vi "5RobotsSkill.vi"(5 "Eliminate":T1, 6 "id":i32, 7 "5Positions":dbl[][](array[numeric]), 8 "error in (no error)":errorcluster, 9 "Robot In":refnum<class "Robot.lvclass">, 10 "Game in":refnum<class "Game.lvclass">, 11 "5RobotsSkill in":refnum<class "5RobotsSkill.lvclass">) -> (0 "error out":errorcluster, 2 "Robot out":refnum<class "Robot.lvclass">, 3 "5RobotsSkill out":refnum<class "5RobotsSkill.lvclass">)   [LabVIEW 2020, in "5RobotsSkill.lvclass"]
uses:
  5RobotsSkill.lvclass
  Game_class/Game.lvclass
  Robot_class/Robot.lvclass
  Ally_class/EliminateEnum.ctl
  Utilities_class/Utilities.lvclass
  Game_class/Game.lvclass/Game.ctl
  Referee_class/Referee.lvclass/Referee.ctl
  Team_class/Team.lvclass/Team.ctl
  Robot_class/Robot.lvclass/Robot.ctl
  d6476285-48f6-47f5-bd76-da5b47b6f033.vi
  b4841ea0-fdbc-4f48-b81d-56e09d8e2016.vi
  0d12ad11-68e3-46b2-a192-4422364186e5.vi
  6660b6ff-d865-414d-86e9-5587d6df92b5.vi
  8726d1a9-8fa9-45be-ba09-7ecc15164713.vi
  Robot_class/Read id.vi
  3b771abe-fd57-4fcc-a3fe-9fcf721aac13.vi
  Team_class/Read RobotRef.vi
  Game_class/Read BallRef.vi
  Game_class/Read Referee.vi
  Referee_class/Read our_goalie_id.vi
  Game_class/Read AllyRef.vi
  Robot_class/Write dest_x.vi
  Robot_class/Write dest_y.vi
  Robot_class/Write dest_orientation.vi
  Robot_class/Write keepDest.vi
  <vilib>/Array/Sort 2D Array - Pop Stack.vi
  <vilib>/Array/Sort 2D Array - Push Stack.vi
  d6476285-48f6-47f5-bd76-da5b47b6f033.vi/269d4b3b-47f5-49e3-8884-44851e4dd9d5.vi
  d6476285-48f6-47f5-bd76-da5b47b6f033.vi/6d99389c-673d-4efb-bf33-19b32bcf4cf8.vi
  b4841ea0-fdbc-4f48-b81d-56e09d8e2016.vi/269d4b3b-47f5-49e3-8884-44851e4dd9d5.vi
  b4841ea0-fdbc-4f48-b81d-56e09d8e2016.vi/6d99389c-673d-4efb-bf33-19b32bcf4cf8.vi
  0d12ad11-68e3-46b2-a192-4422364186e5.vi/269d4b3b-47f5-49e3-8884-44851e4dd9d5.vi
  0d12ad11-68e3-46b2-a192-4422364186e5.vi/6d99389c-673d-4efb-bf33-19b32bcf4cf8.vi
  6660b6ff-d865-414d-86e9-5587d6df92b5.vi/269d4b3b-47f5-49e3-8884-44851e4dd9d5.vi
  6660b6ff-d865-414d-86e9-5587d6df92b5.vi/6d99389c-673d-4efb-bf33-19b32bcf4cf8.vi
  8726d1a9-8fa9-45be-ba09-7ecc15164713.vi/269d4b3b-47f5-49e3-8884-44851e4dd9d5.vi
  8726d1a9-8fa9-45be-ba09-7ecc15164713.vi/6d99389c-673d-4efb-bf33-19b32bcf4cf8.vi
  Ally_class/Ally.lvclass
  C:/Users/anton/Desktop/RoboIME/SSL_COMP/SSL_AI/Team_class/Team.lvclass
  Ball_class/Ball.lvclass
  Referee_class/Referee.lvclass
  <vilib>/Comparison/Less/Less Functor/Less Functor.lvclass
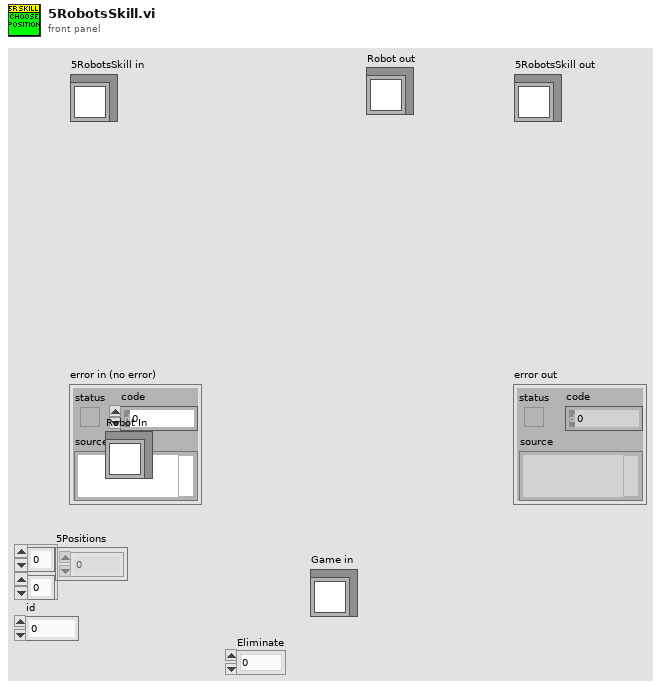
[diagram p1: front panel]
types:
  T1 = typedef "EliminateEnum.ctl" = enum16{"0", "1", "2"}
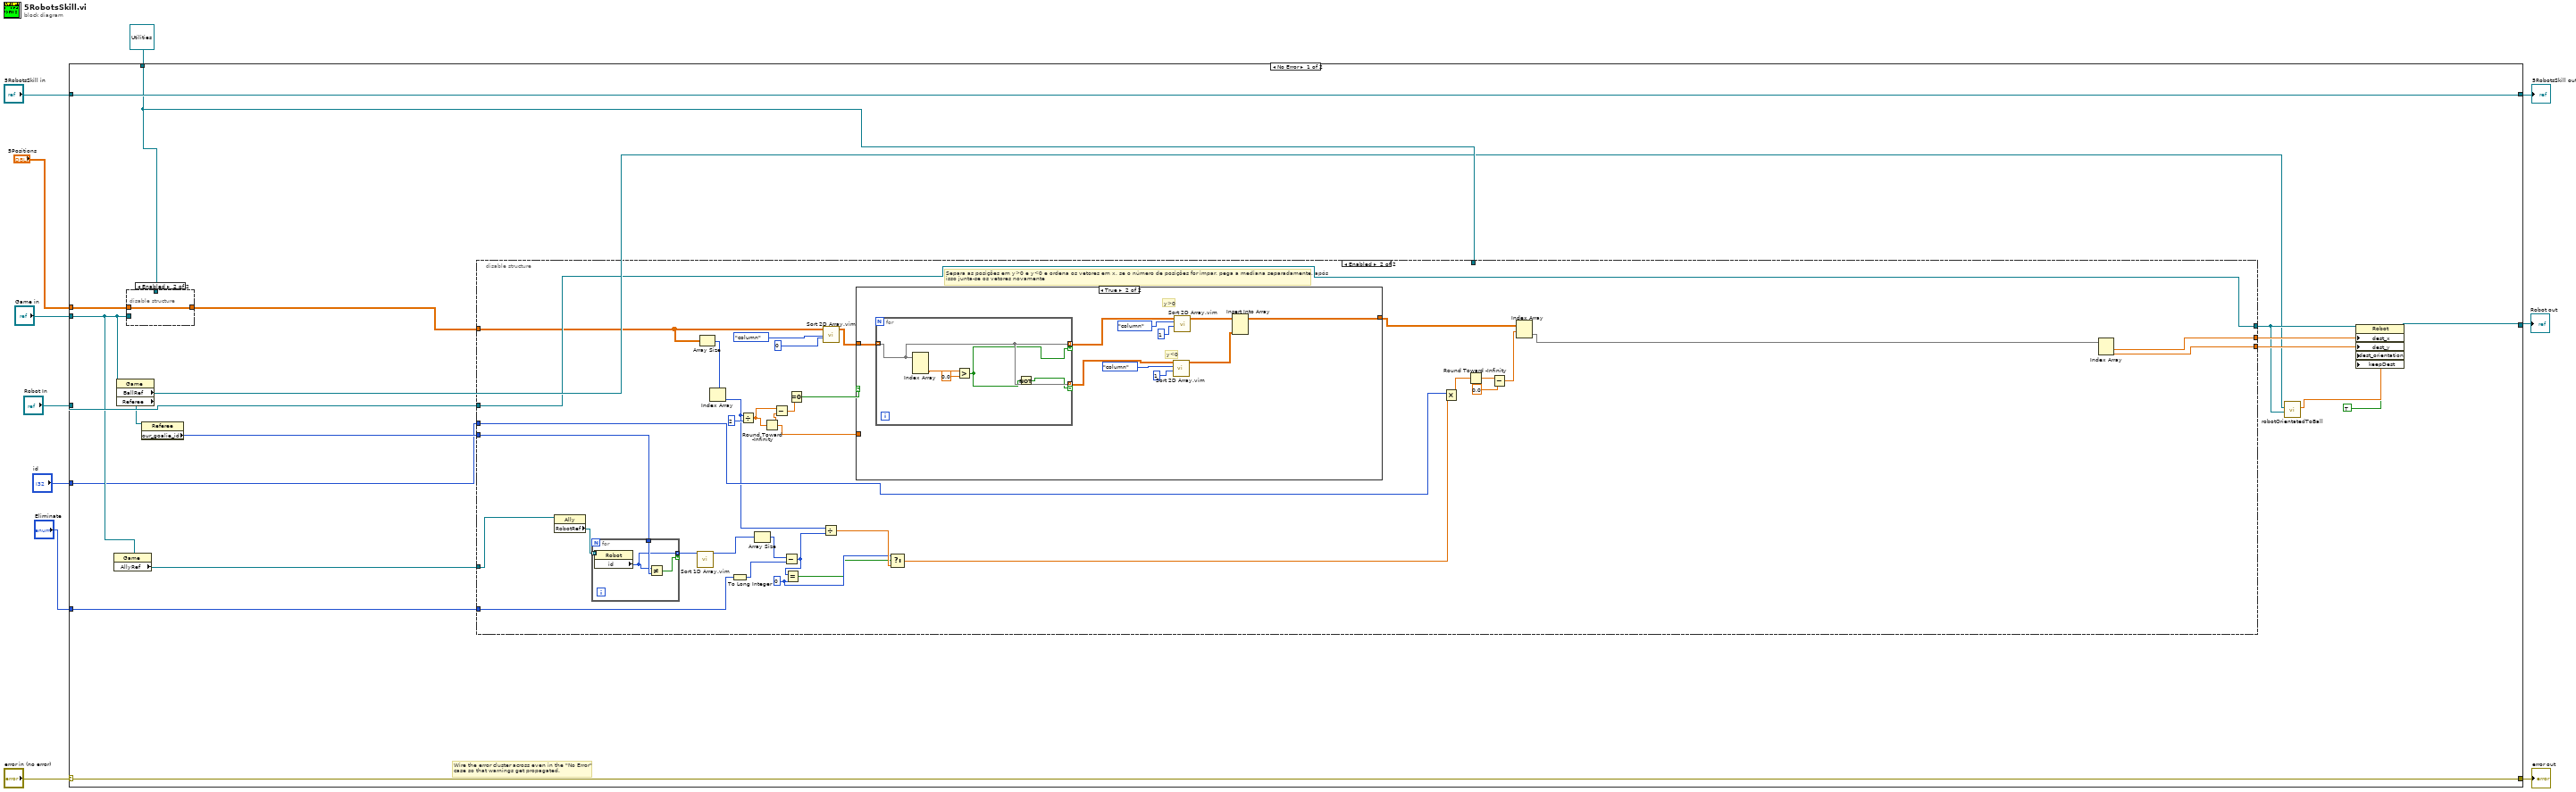
[diagram p0: block diagram]
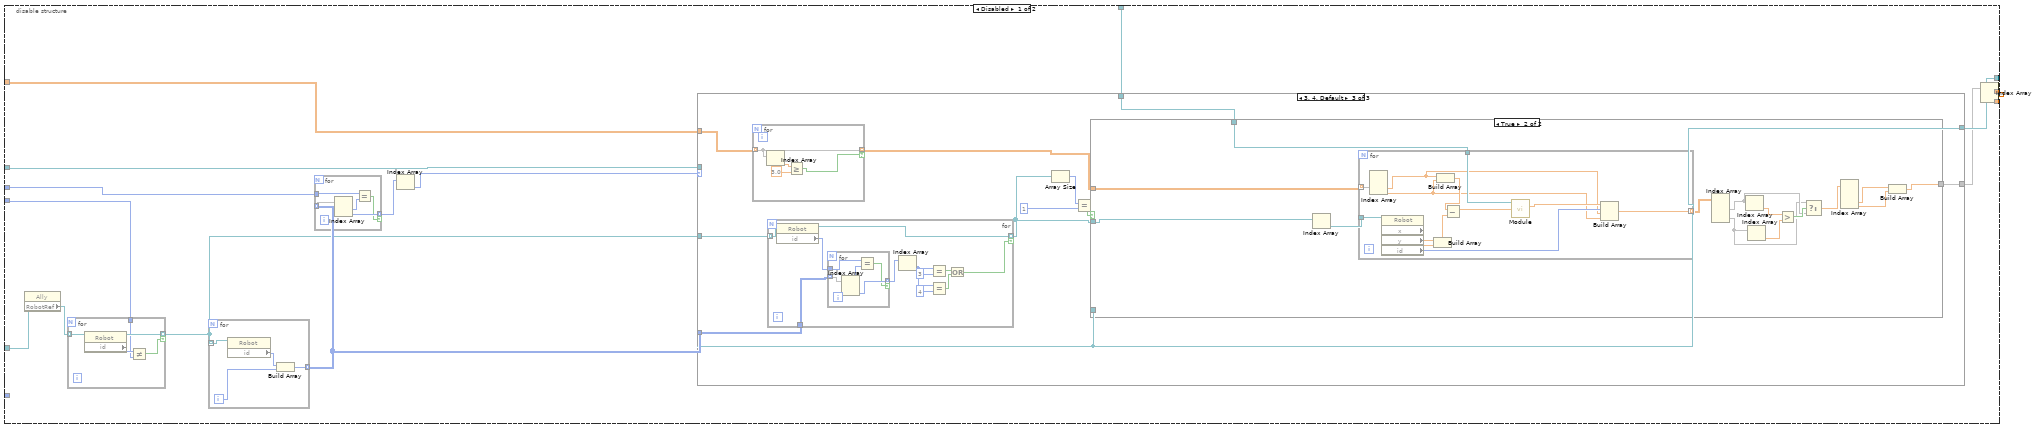
[diagram p2: hidden frame]
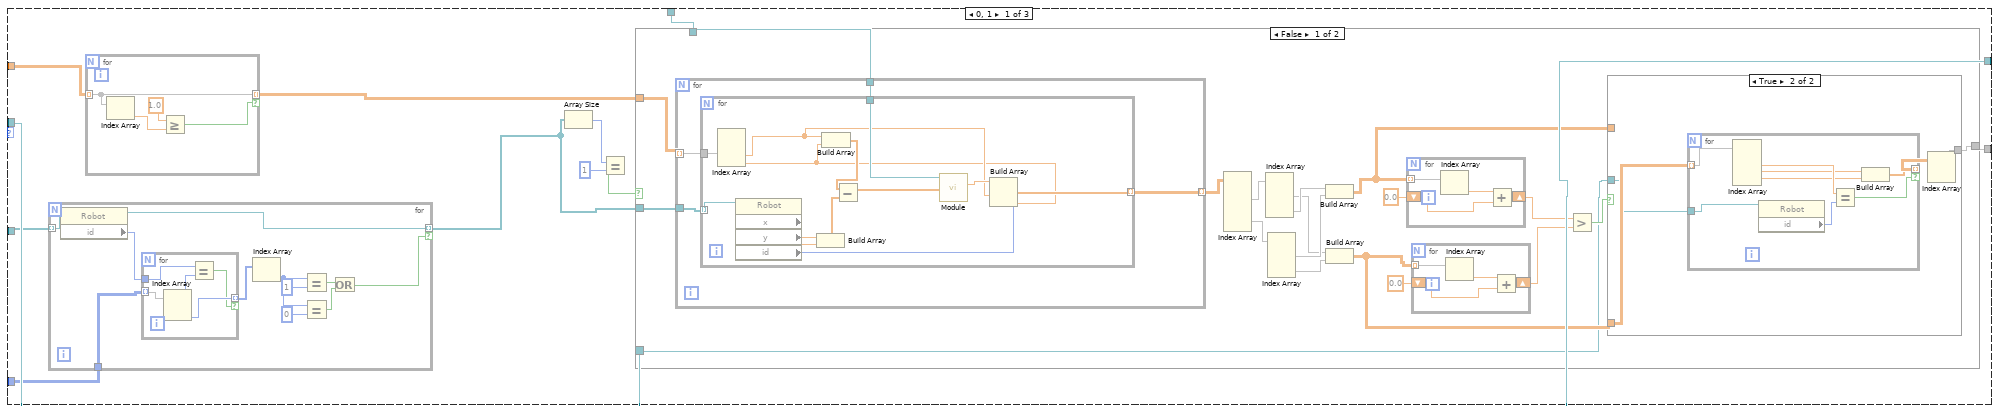
[diagram p3: hidden frame]
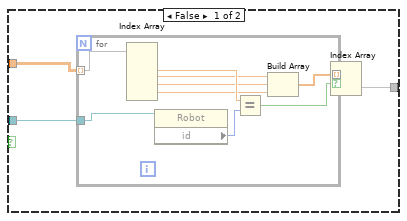
[diagram p4: hidden frame]
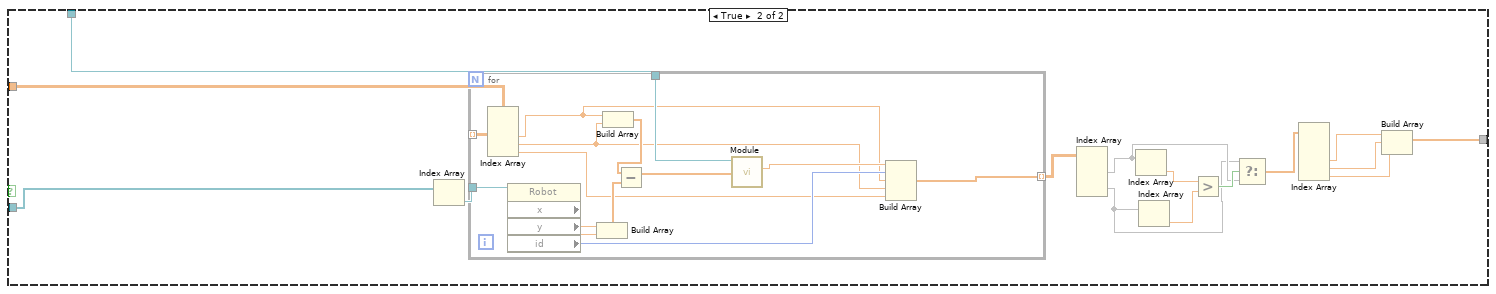
[diagram p5: hidden frame]
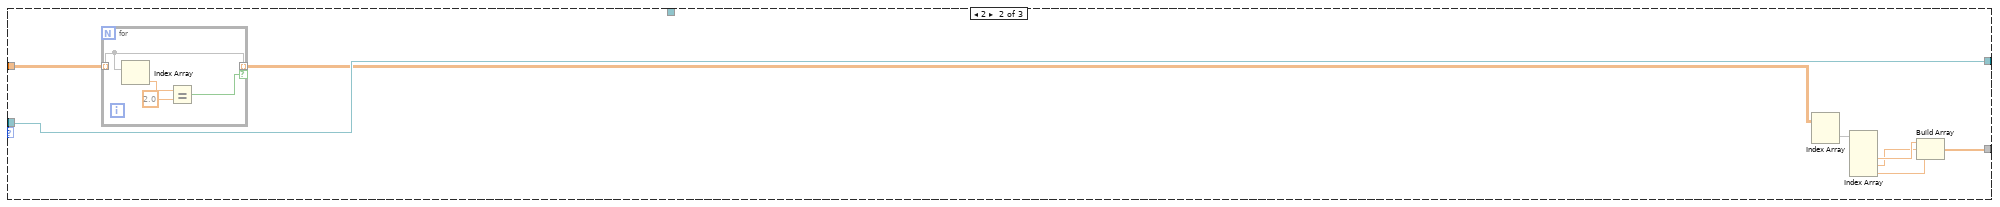
[diagram p6: hidden frame]
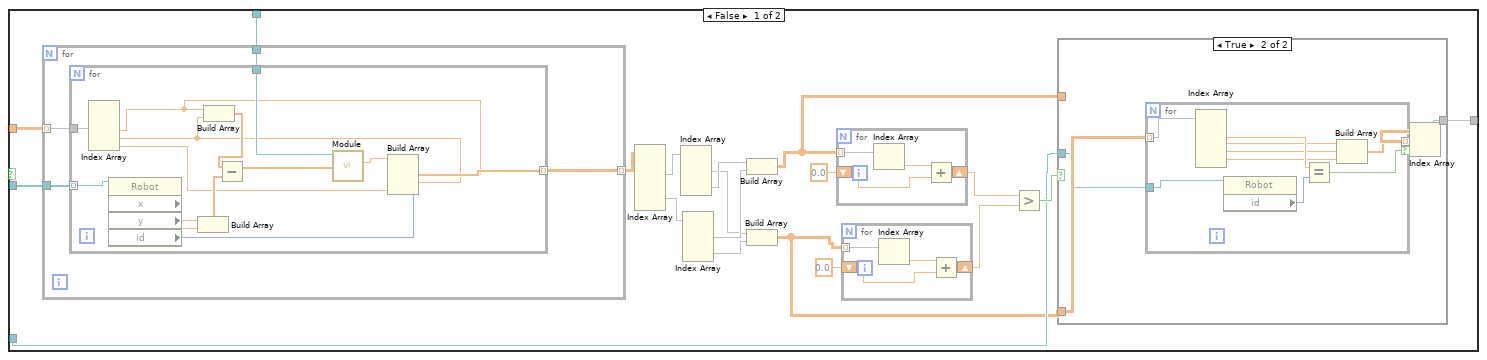
[diagram p7: hidden frame]
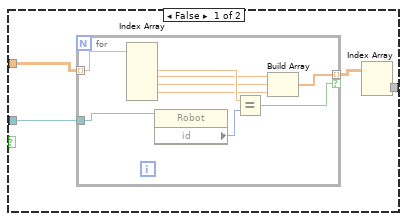
[diagram p8: hidden frame]
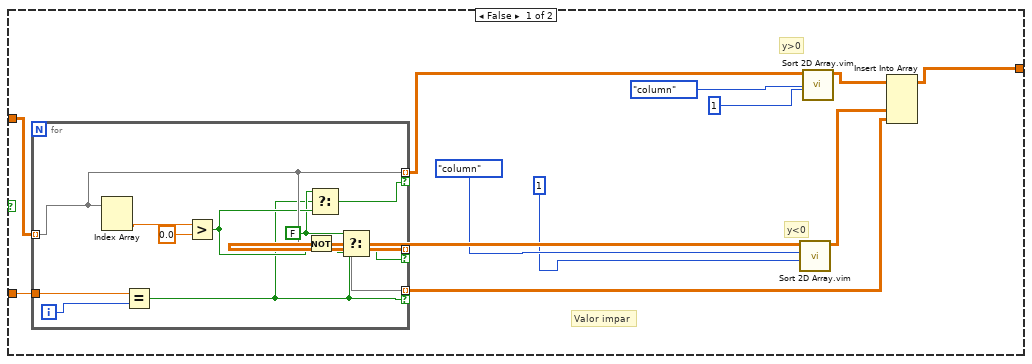
[diagram p9: hidden frame]
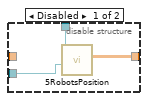
[diagram p10: hidden frame]
diagram:
  n1 = case shown="No Error" "error in (no error)" {
    selector: "error in (no error)" -> [w29 w412]
    tunnel: [w29 w412] -> w10
    tunnel: [w30 w411] -> w8
    tunnel: "5RobotsSkill in" -> [w30 w411]
    tunnel: refnum<class "Utilities.lvclass"> refnum ("Utilities in") -> [w27 _]
    tunnel: "Game in" -> [w21 _]
    tunnel: "Robot In" -> [w28 w410]
    tunnel: [w26 w410] -> w4
    tunnel: "5Positions" -> [w19 _]
    tunnel: "id" -> [w13 _]
    tunnel: "Eliminate" -> [w12 _]
    frame No Error {
      # "Wire the error cluster across even in the \"No Error\"\ncase so that warnings get propagated."
      n2 = property class="Game"(reference=w21) -> ("AllyRef"=w17:refnum<class "Ally.lvclass">)  [unwired: 1 in, 2 out]
      n3 = property class="Game"(reference=w21) -> ("BallRef"=w20:refnum<class "Ball.lvclass">, "Referee"=w16:refnum<class "Referee.lvclass">)  [unwired: 1 in, 2 out]
      n4 = disable-structure shown="Enabled" {
        disable-tunnel: [w408 w409] -> w14
        disable-tunnel: w27 -> [w407 _]
        disable-tunnel: w21 -> [w406 _]
        disable-tunnel: w19 -> [_ w409]
        frame Disabled {
          n5 = call-dynamic "5RobotsPosition.vi"("Game"=w406, "Utilities in"=w407) -> ("5Positions"=w408:dbl[][])  [unwired: 7 in, 2 out]
        }
        frame Enabled {
        }
      }
      n6 = property class="Referee"(reference=w16) -> ("our_goalie_id"=w15:i32)  [unwired: 1 in, 2 out]
      n7 = disable-structure shown="Enabled" {
        disable-tunnel: w28 -> [w45 w344]
        disable-tunnel: w27 -> [w44 _]
        disable-tunnel: [w43 w338] -> w24
        disable-tunnel: [w42 w343] -> w23
        disable-tunnel: [w41 w344] -> w22
        disable-tunnel: w17 -> [w40 w362]
        disable-tunnel: w13 -> [w38 w351]
        disable-tunnel: w15 -> [w33 w361]
        disable-tunnel: w14 -> [w32 w340]
        disable-tunnel: w12 -> [_ w333]
        frame Disabled {
          n8 = property class="Ally"(reference=w40) -> ("RobotRef"=w34:refnum<class "Robot.lvclass">[])  [unwired: 1 in, 2 out]
          n9 = for {
            tunnel: w34 -> [w320] mode=indexing
            tunnel: [w319] -> w31 mode=indexing if=w317
            tunnel: w33 -> [w316]
            n10 = property class="Robot"(reference=w320) -> (reference out=w319:refnum<class "Robot.lvclass">, "id"=w318:i32)  [unwired: 1 in, 1 out]
            n11 = Not Equal?(x=w318, y=w316) -> (x != y?=w317:bool)
          }
          n12 = for {
            tunnel: w31 -> [w329] mode=indexing
            tunnel: [w327] -> w35 mode=indexing
            i -> [w326]
            n13 = property class="Robot"(reference=w329) -> ("id"=w328:i32)  [unwired: 1 in, 2 out]
            n14 = Build Array(w328, w326) -> (w327:i32[])
          }
          n15 = for {
            tunnel: w38 -> [w322]
            tunnel: w35 -> [w325] mode=indexing
            tunnel: [w324] -> w36 mode=indexing if=w321
            n16 = Index Array(array=w325) -> (element #1=w323:i32, element #2=w324:i32)  [unwired: 2 in]
            n17 = Equal?(x=w322, y=w323) -> (x = y?=w321:bool)
          }
          n18 = Index Array(array=w36) -> (element=w37:i32)  [unwired: 1 in]
          n19 = case shown="3, 4, Default" w37 {
            tunnel: w44 -> [w56 _ w196]
            tunnel: w45 -> [w54 w181 w194]
            tunnel: w32 -> [w50 w182 w197]
            tunnel: [w55 w176 w195] -> w39
            tunnel: [w54 w181 w194] -> w41
            tunnel: w31 -> [w48 _ w188]
            tunnel: w35 -> [w47 _ w187]
            frame 0, 1 {
              n20 = for {
                tunnel: [w165] -> w46 mode=indexing if=w155
                tunnel: w48 -> [w164] mode=indexing
                tunnel: w47 -> [w162]
                n21 = property class="Robot"(reference=w164) -> (reference out=w165:refnum<class "Robot.lvclass">, "id"=w163:i32)  [unwired: 1 in, 1 out]
                n22 = for {
                  tunnel: w163 -> [w169]
                  tunnel: w162 -> [w170] mode=indexing
                  tunnel: [w167] -> w161 mode=indexing if=w166
                  n23 = Index Array(array=w170) -> (element #1=w168:i32, element #2=w167:i32)  [unwired: 2 in]
                  n24 = Equal?(x=w169, y=w168) -> (x = y?=w166:bool)
                }
                n25 = Index Array(array=w161) -> (element=w160:i32)  [unwired: 1 in]
                n26 = Equal?(x=w160, y=1) -> (x = y?=w157:bool)
                n27 = Equal?(x=w160, y=0) -> (x = y?=w156:bool)
                n28 = Or(x=w157, y=w156) -> (x .or. y?=w155:bool)
              }
              n29 = for {
                tunnel: w50 -> [w174] mode=indexing
                tunnel: [w174] -> w49 mode=indexing if=w173
                n30 = Index Array(array=w174) -> (element=w171:dbl)  [unwired: 1 in]
                n31 = Greater Or Equal?(x=1.0 ("y"), y=w171) -> (x >= y?=w173:bool)
              }
              n32 = Array Size(array=w46) -> (size(s)=w51:i32)
              n33 = Equal?(x=w51, y=1) -> (x = y?=w53:bool)
              n34 = case shown="False" w53 {
                tunnel: w46 -> [w75 w138]
                tunnel: w56 -> [w74 w136]
                tunnel: w49 -> [w73 w139]
                tunnel: [w57 w140] -> w55
                tunnel: w54 -> [w58 _]
                frame False {
                  n35 = for {
                    tunnel: w75 -> [w112]
                    tunnel: w74 -> [w111]
                    tunnel: w73 -> [w110] mode=indexing
                    tunnel: [w109] -> w59 mode=indexing
                    n36 = for {
                      tunnel: w112 -> [w125] mode=indexing
                      tunnel: w110 -> [w117]
                      tunnel: w111 -> [w120]
                      tunnel: [w119] -> w109 mode=indexing
                      n37 = Index Array(array=w117) -> (element #2=w114:dbl, element #3=w113:dbl)  [unwired: 3 in, 1 out]
                      n38 = property class="Robot"(reference=w125) -> ("x"=w124:dbl, "y"=w123:dbl, "id"=w116:i32)  [unwired: 1 in, 2 out]
                      n39 = Build Array(w124, w123) -> (w122:dbl[])
                      n40 = Build Array(w114, w113) -> (w115:dbl[])
                      n41 = Subtract(x=w115, y=w122) -> (x-y=w121:dbl[])
                      n42 = call "Module.vi"("2D vector"=w121, "Utilities in"=w120) -> ("Modulo"=w118:dbl)  [unwired: 7 in, 2 out]
                      n43 = Build Array(w118, w116, w114, w113) -> (w119:dbl[])
                    }
                  }
                  n44 = Index Array(array=w59) -> (element #1=w67:dbl[][], element #2=w66:dbl[][])  [unwired: 6 in]
                  n45 = Index Array(array=w67) -> (element #1=w63:dbl[], element #2=w64:dbl[])  [unwired: 4 in]
                  n46 = Index Array(array=w66) -> (element #1=w65:dbl[], element #2=w62:dbl[])  [unwired: 4 in]
                  n47 = Build Array(w64, w65) -> (w60:dbl[][])
                  n48 = Build Array(w63, w62) -> (w61:dbl[][])
                  n49 = for {
                    tunnel: w60 -> [w108] mode=indexing
                    shift-right: [w106] -> w70
                    shift-left: 0.0 -> [w105]
                    n50 = Index Array(array=w108) -> (element=w107:dbl)  [unwired: 1 in]
                    n51 = Add(x=w107, y=w105) -> (x+y=w106:dbl)
                  }
                  n52 = for {
                    tunnel: w61 -> [w104] mode=indexing
                    shift-right: [w102] -> w69
                    shift-left: 0.0 -> [w101]
                    n53 = Index Array(array=w104) -> (element=w103:dbl)  [unwired: 1 in]
                    n54 = Add(x=w103, y=w101) -> (x+y=w102:dbl)
                  }
                  n55 = Greater?(x=w70, y=w69) -> (0:w68:bool)
                  n56 = case shown="True" w68 {
                    tunnel: w60 -> [w79 _]
                    tunnel: w61 -> [_ w90]
                    tunnel: w58 -> [w78 w89]
                    tunnel: [w76 w91] -> w57
                    frame False {
                      n57 = for {
                        tunnel: w79 -> [w87] mode=indexing
                        tunnel: w78 -> [w88]
                        tunnel: [w81] -> w77 mode=indexing if=w80
                        n58 = Index Array(array=w87) -> (element #2=w85:dbl, element #3=w84:dbl, element #4=w83:dbl, element #5=w82:dbl)  [unwired: 5 in, 1 out]
                        n59 = property class="Robot"(reference=w88) -> ("id"=w86:i32)  [unwired: 1 in, 2 out]
                        n60 = Equal?(x=w85, y=w86) -> (x = y?=w80:bool)
                        n61 = Build Array(w84, w83, w82) -> (w81:dbl[])
                      }
                      n62 = Index Array(array=w77) -> (element=w76:dbl[])  [unwired: 2 in]
                    }
                    frame True {
                      n63 = for {
                        tunnel: w90 -> [w99] mode=indexing
                        tunnel: w89 -> [w100]
                        tunnel: [w94] -> w92 mode=indexing if=w93
                        n64 = Index Array(array=w99) -> (element #2=w97:dbl, element #3=w96:dbl, element #4=w95:dbl)  [unwired: 4 in, 1 out]
                        n65 = property class="Robot"(reference=w100) -> ("id"=w98:i32)  [unwired: 1 in, 2 out]
                        n66 = Equal?(x=w97, y=w98) -> (x = y?=w93:bool)
                        n67 = Build Array(w96, w95) -> (w94:dbl[])
                      }
                      n68 = Index Array(array=w92) -> (element=w91:dbl[])  [unwired: 2 in]
                    }
                  }
                }
                frame True {
                  n69 = Index Array(array=w138) -> (element=w137:refnum<class "Robot.lvclass">)  [unwired: 1 in]
                  n70 = for {
                    tunnel: w139 -> [w147] mode=indexing
                    tunnel: w136 -> [w150]
                    tunnel: [w149] -> w135 mode=indexing
                    tunnel: w137 -> [w141]
                    n71 = Index Array(array=w147) -> (element #2=w144:dbl, element #3=w143:dbl, element #4=w142:dbl)  [unwired: 4 in, 1 out]
                    n72 = property class="Robot"(reference=w141) -> ("x"=w154:dbl, "y"=w153:dbl, "id"=w146:i32)  [unwired: 1 in, 2 out]
                    n73 = Build Array(w154, w153) -> (w152:dbl[])
                    n74 = Build Array(w144, w143) -> (w145:dbl[])
                    n75 = Subtract(x=w145, y=w152) -> (x-y=w151:dbl[])
                    n76 = call "Module.vi"("2D vector"=w151, "Utilities in"=w150) -> ("Modulo"=w148:dbl)  [unwired: 7 in, 2 out]
                    n77 = Build Array(w148, w146, w144, w143, w142) -> (w149:dbl[])
                  }
                  n78 = Index Array(array=w135) -> (element #1=w131:dbl[], element #2=w130:dbl[])  [unwired: 4 in]
                  n79 = Index Array(array=w131) -> (element=w134:dbl)  [unwired: 1 in]
                  n80 = Index Array(array=w130) -> (element=w133:dbl)  [unwired: 1 in]
                  n81 = Greater?(x=w134, y=w133) -> (0:w132:bool)
                  n82 = Select(t=w130, s=w132, f=w131) -> (s? t:f=w129:dbl[])
                  n83 = Index Array(array=w129) -> (element #3=w128:dbl, element #4=w127:dbl, element #5=w126:dbl)  [unwired: 5 in, 2 out]
                  n84 = Build Array(w128, w127, w126) -> (w140:dbl[])
                }
              }
            }
            frame 2 {
              n85 = for {
                tunnel: w182 -> [w185] mode=indexing
                tunnel: [w185] -> w175 mode=indexing if=w186
                n86 = Index Array(array=w185) -> (element=w184:dbl)  [unwired: 1 in]
                n87 = Equal?(x=w184, y=2.0) -> (x = y?=w186:bool)
              }
              n88 = Index Array(array=w175) -> (element=w180:dbl[])  [unwired: 2 in]
              n89 = Index Array(array=w180) -> (element #2=w179:dbl, element #3=w178:dbl, element #4=w177:dbl)  [unwired: 4 in, 1 out]
              n90 = Build Array(w179, w178, w177) -> (w176:dbl[])
            }
            frame 3, 4, Default {
              n91 = for {
                tunnel: w197 -> [w315] mode=indexing
                tunnel: [w315] -> w191 mode=indexing if=w314
                n92 = Index Array(array=w315) -> (element=w312:dbl)  [unwired: 1 in]
                n93 = Greater Or Equal?(x=w312, y=3.0) -> (x >= y?=w314:bool)
              }
              n94 = for {
                tunnel: [w306] -> w189 mode=indexing if=w296
                tunnel: w188 -> [w305] mode=indexing
                tunnel: w187 -> [w303]
                n95 = property class="Robot"(reference=w305) -> (reference out=w306:refnum<class "Robot.lvclass">, "id"=w304:i32)  [unwired: 1 in, 1 out]
                n96 = for {
                  tunnel: w304 -> [w310]
                  tunnel: w303 -> [w311] mode=indexing
                  tunnel: [w308] -> w302 mode=indexing if=w307
                  n97 = Index Array(array=w311) -> (element #1=w309:i32, element #2=w308:i32)  [unwired: 2 in]
                  n98 = Equal?(x=w310, y=w309) -> (x = y?=w307:bool)
                }
                n99 = Index Array(array=w302) -> (element=w301:i32)  [unwired: 1 in]
                n100 = Equal?(x=w301, y=3) -> (x = y?=w298:bool)
                n101 = Equal?(x=w301, y=4) -> (x = y?=w297:bool)
                n102 = Or(x=w298, y=w297) -> (x .or. y?=w296:bool)
              }
              n103 = Array Size(array=w189) -> (size(s)=w190:i32)
              n104 = Equal?(x=w190, y=1) -> (x = y?=w192:bool)
              n105 = case shown="True" w192 {
                tunnel: w196 -> [w216 w270]
                tunnel: w191 -> [w215 w271]
                tunnel: [w208 w272] -> w195
                tunnel: w194 -> [w207 _]
                tunnel: w189 -> [w198 w269]
                frame False {
                  n106 = for {
                    tunnel: w216 -> [w254]
                    tunnel: w215 -> [w253] mode=indexing
                    tunnel: [w252] -> w214 mode=indexing
                    tunnel: w198 -> [w251]
                    n107 = for {
                      tunnel: w253 -> [w261]
                      tunnel: w254 -> [w264]
                      tunnel: [w263] -> w252 mode=indexing
                      tunnel: w251 -> [w255] mode=indexing
                      n108 = Index Array(array=w261) -> (element #2=w258:dbl, element #3=w257:dbl, element #4=w256:dbl)  [unwired: 4 in, 1 out]
                      n109 = property class="Robot"(reference=w255) -> ("x"=w268:dbl, "y"=w267:dbl, "id"=w260:i32)  [unwired: 1 in, 2 out]
                      n110 = Build Array(w268, w267) -> (w266:dbl[])
                      n111 = Build Array(w258, w257) -> (w259:dbl[])
                      n112 = Subtract(x=w259, y=w266) -> (x-y=w265:dbl[])
                      n113 = call "Module.vi"("2D vector"=w265, "Utilities in"=w264) -> ("Modulo"=w262:dbl)  [unwired: 7 in, 2 out]
                      n114 = Build Array(w262, w260, w258, w257, w256) -> (w263:dbl[])
                    }
                  }
                  n115 = Index Array(array=w214) -> (element #1=w206:dbl[][], element #2=w205:dbl[][])  [unwired: 6 in]
                  n116 = Index Array(array=w206) -> (element #1=w202:dbl[], element #2=w203:dbl[])  [unwired: 4 in]
                  n117 = Index Array(array=w205) -> (element #1=w204:dbl[], element #2=w201:dbl[])  [unwired: 4 in]
                  n118 = Build Array(w203, w204) -> (w199:dbl[][])
                  n119 = Build Array(w202, w201) -> (w200:dbl[][])
                  n120 = for {
                    tunnel: w199 -> [w250] mode=indexing
                    shift-right: [w248] -> w211
                    shift-left: 0.0 -> [w247]
                    n121 = Index Array(array=w250) -> (element=w249:dbl)  [unwired: 1 in]
                    n122 = Add(x=w249, y=w247) -> (x+y=w248:dbl)
                  }
                  n123 = for {
                    tunnel: w200 -> [w246] mode=indexing
                    shift-right: [w244] -> w210
                    shift-left: 0.0 -> [w243]
                    n124 = Index Array(array=w246) -> (element=w245:dbl)  [unwired: 1 in]
                    n125 = Add(x=w245, y=w243) -> (x+y=w244:dbl)
                  }
                  n126 = Greater?(x=w211, y=w210) -> (0:w209:bool)
                  n127 = case shown="True" w209 {
                    tunnel: w199 -> [w220 _]
                    tunnel: w200 -> [_ w231]
                    tunnel: w207 -> [w219 w230]
                    tunnel: [w217 w232] -> w208
                    frame False {
                      n128 = for {
                        tunnel: w220 -> [w228] mode=indexing
                        tunnel: w219 -> [w229]
                        tunnel: [w222] -> w218 mode=indexing if=w221
                        n129 = Index Array(array=w228) -> (element #2=w226:dbl, element #3=w225:dbl, element #4=w224:dbl, element #5=w223:dbl)  [unwired: 5 in, 1 out]
                        n130 = property class="Robot"(reference=w229) -> ("id"=w227:i32)  [unwired: 1 in, 2 out]
                        n131 = Equal?(x=w226, y=w227) -> (x = y?=w221:bool)
                        n132 = Build Array(w225, w224, w223) -> (w222:dbl[])
                      }
                      n133 = Index Array(array=w218) -> (element=w217:dbl[])  [unwired: 2 in]
                    }
                    frame True {
                      n134 = for {
                        tunnel: w231 -> [w241] mode=indexing
                        tunnel: w230 -> [w242]
                        tunnel: [w235] -> w233 mode=indexing if=w234
                        n135 = Index Array(array=w241) -> (element #2=w239:dbl, element #3=w238:dbl, element #4=w237:dbl, element #5=w236:dbl)  [unwired: 5 in, 1 out]
                        n136 = property class="Robot"(reference=w242) -> ("id"=w240:i32)  [unwired: 1 in, 2 out]
                        n137 = Equal?(x=w239, y=w240) -> (x = y?=w234:bool)
                        n138 = Build Array(w238, w237, w236) -> (w235:dbl[])
                      }
                      n139 = Index Array(array=w233) -> (element=w232:dbl[])  [unwired: 2 in]
                    }
                  }
                }
                frame True {
                  n140 = Index Array(array=w269) -> (element=w282:refnum<class "Robot.lvclass">)  [unwired: 1 in]
                  n141 = for {
                    tunnel: w271 -> [w288] mode=indexing
                    tunnel: w270 -> [w291]
                    tunnel: [w290] -> w281 mode=indexing
                    tunnel: w282 -> [w283]
                    n142 = Index Array(array=w288) -> (element #2=w285:dbl, element #3=w284:dbl)  [unwired: 3 in, 1 out]
                    n143 = property class="Robot"(reference=w283) -> ("x"=w295:dbl, "y"=w294:dbl, "id"=w287:i32)  [unwired: 1 in, 2 out]
                    n144 = Build Array(w295, w294) -> (w293:dbl[])
                    n145 = Build Array(w285, w284) -> (w286:dbl[])
                    n146 = Subtract(x=w286, y=w293) -> (x-y=w292:dbl[])
                    n147 = call "Module.vi"("2D vector"=w292, "Utilities in"=w291) -> ("Modulo"=w289:dbl)  [unwired: 7 in, 2 out]
                    n148 = Build Array(w289, w287, w285, w284) -> (w290:dbl[])
                  }
                  n149 = Index Array(array=w281) -> (element #1=w277:dbl[], element #2=w276:dbl[])  [unwired: 4 in]
                  n150 = Index Array(array=w277) -> (element=w280:dbl)  [unwired: 1 in]
                  n151 = Index Array(array=w276) -> (element=w279:dbl)  [unwired: 1 in]
                  n152 = Greater?(x=w280, y=w279) -> (0:w278:bool)
                  n153 = Select(t=w276, s=w278, f=w277) -> (s? t:f=w275:dbl[])
                  n154 = Index Array(array=w275) -> (element #3=w274:dbl, element #4=w273:dbl)  [unwired: 4 in, 2 out]
                  n155 = Build Array(w274, w273) -> (w272:dbl[])
                }
              }
            }
          }
          n156 = Index Array(array=w39) -> (element #1=w43:dbl, element #2=w42:dbl)  [unwired: 2 in]
        }
        frame Enabled {
          w336 = 0 ("y")
          # "Separa as posições em y>0 e y<0 e ordena os vetores em x, se o número de posições for impar, pega a mediana separadamente, após \nisso junta-se os vetores novamente"
          n157 = property class="Ally"(reference=w362) -> ("RobotRef"=w363:refnum<class "Robot.lvclass">[])  [unwired: 1 in, 2 out]
          n158 = for {
            tunnel: w363 -> [w405] mode=indexing
            tunnel: [w402] -> w360 mode=indexing if=w404
            tunnel: w361 -> [w403]
            n159 = property class="Robot"(reference=w405) -> ("id"=w402:i32)  [unwired: 1 in, 2 out]
            n160 = Not Equal?(x=w402, y=w403) -> (x != y?=w404:bool)
          }
          n161 = call "Sort 1D Array.vim"("unsorted array"=w360) -> ("sorted array"=w359:i32[])  [unwired: 10 in]
          n162 = Array Size(array=w340) -> (size(s)=w358:i32[])
          n163 = Index Array(array=w358) -> (element=w346:i32)  [unwired: 1 in]
          n164 = To Long Integer(number=w333) -> (32bit integer=w332:i32)
          n165 = Divide(x=w346, y=2) -> (x/y=w347:dbl)
          n166 = Array Size(array=w359) -> (size(s)=w334:i32)
          n167 = Round Toward -Infinity(1:w347) -> (0:w354:dbl)
          n168 = Subtract(x=w347, y=w354) -> (x-y=w355:dbl)
          n169 = Subtract(x=w334, y=w332) -> (x-y=w331:i32)
          n170 = Equal?(x=w331, y=w336) -> (x = y?=w330:bool)
          n171 = Equal To 0?(x=w355) -> (x = 0?=w356:bool)
          n172 = Divide(x=w346, y=w331) -> (x/y=w337:dbl)
          n173 = call "Sort 2D Array.vim"("index"=0, "dimension to index (column)"=enum16{"column", "row"}."column", "2D array"=w340) -> ("sorted 2D array"=w339:dbl[][])  [unwired: 7 in, 1 out]
          n174 = case shown="True" w356 {
            tunnel: w354 -> [w369 _]
            tunnel: [w367 w390] -> w353
            tunnel: w339 -> [w364 w387]
            frame False {
              # "Valor impar"
              # "y<0"
              # "y>0"
              n175 = for {
                tunnel: w364 -> [w383] mode=indexing
                tunnel: [w383] -> w375 mode=indexing if=w381
                tunnel: [w383] -> w374 mode=indexing if=w378
                tunnel: [w383] -> w365 mode=indexing if=w377
                tunnel: w369 -> [w376]
                i -> [w384]
                w379 = FALSE ("t")
                n176 = Index Array(array=w383) -> (element #2=w385:dbl)  [unwired: 2 in, 1 out]
                n177 = Equal?(x=w376, y=w384) -> (x = y?=w377:bool)
                n178 = Greater?(x=w385, y=0.0) -> (0:w380:bool)
                n179 = Not(x=w380) -> (.not. x?=w382:bool)
                n180 = Select(t=w379, s=w377, f=w380) -> (s? t:f=w381:bool)
                n181 = Select(t=w379, s=w377, f=w382) -> (s? t:f=w378:bool)
              }
              n182 = call "Sort 2D Array.vim"("index"=1, "dimension to index (column)"=enum16{"column", "row"}."column", "2D array"=w374) -> ("sorted 2D array"=w366:dbl[][])  [unwired: 7 in, 1 out]
              n183 = call "Sort 2D Array.vim"("index"=1, "dimension to index (column)"=enum16{"column", "row"}."column", "2D array"=w375) -> ("sorted 2D array"=w368:dbl[][])  [unwired: 7 in, 1 out]
              n184 = Insert Into Array(array=w368, new element #1=w366, new element #2=w365) -> (w367:dbl[][])  [unwired: 2 in]
            }
            frame True {
              # "y<0"
              # "y>0"
              n185 = for {
                tunnel: w387 -> [w399] mode=indexing
                tunnel: [w399] -> w392 mode=indexing if=w397
                tunnel: [w399] -> w389 mode=indexing if=w398
                n186 = Index Array(array=w399) -> (element #3=w400:dbl)  [unwired: 3 in, 2 out]
                n187 = Greater?(x=w400, y=0.0) -> (0:w397:bool)
                n188 = Not(x=w397) -> (.not. x?=w398:bool)
              }
              n189 = call "Sort 2D Array.vim"("index"=1, "dimension to index (column)"=enum16{"column", "row"}."column", "2D array"=w389) -> ("sorted 2D array"=w388:dbl[][])  [unwired: 7 in, 1 out]
              n190 = call "Sort 2D Array.vim"("index"=1, "dimension to index (column)"=enum16{"column", "row"}."column", "2D array"=w392) -> ("sorted 2D array"=w391:dbl[][])  [unwired: 7 in, 1 out]
              n191 = Insert Into Array(array=w391, new element=w388) -> (w390:dbl[][])  [unwired: 2 in]
            }
          }
          n192 = Select(t=w336, s=w330, f=w337) -> (s? t:f=w335:dbl)
          n193 = Multiply(x=w351, y=w335) -> (x*y=w352:dbl)
          n194 = Round Toward -Infinity(1:w352) -> (0:w350:dbl)
          n195 = Subtract(x=w350, y=0.0) -> (x-y=w348:dbl)
          n196 = Index Array(array=w353, index (row)=w348) -> (element=w345:dbl[])  [unwired: 1 in]
          n197 = Index Array(array=w345) -> (element #1=w338:dbl, element #2=w343:dbl)  [unwired: 2 in]
        }
      }
      n198 = call "robotOrientatedToBall.vi"("Robot"=w22, "BallRef"=w20) -> ("Orientation"=w25:dbl)  [unwired: 7 in, 2 out]
      n199 = property class="Robot"(reference=w22, "dest_x"=w24, "dest_y"=w23, "dest_orientation"=w25, "keepDest"=TRUE) -> (reference out=w26:refnum<class "Robot.lvclass">)  [unwired: 1 in, 1 out]
    }
    frame Error {
    }
  }
  "error out" <- w10
  "5RobotsSkill out" <- w8
  "Robot out" <- w4
